vi "Add State to Macro.vi"(5 "Before or After? (Before)":T1, 7 "Before (or After) State":string, 8 "error in (no error)":errorcluster, 9 "State to Add":string, 10 "Macro Name":string, 11 "JKI SM in":refnum<class "JKI SM.lvclass">) -> (0 "error out":errorcluster, 3 "JKI SM out":refnum<class "JKI SM.lvclass">)   [LabVIEW 2013, in "JKI State Machine API.lvlib" / "JKI SM.lvclass"]
uses:
  JKI SM.lvclass
  Typedefs/Before or After -- Enum.ctl
  JKI SM.lvclass/JKI SM.ctl
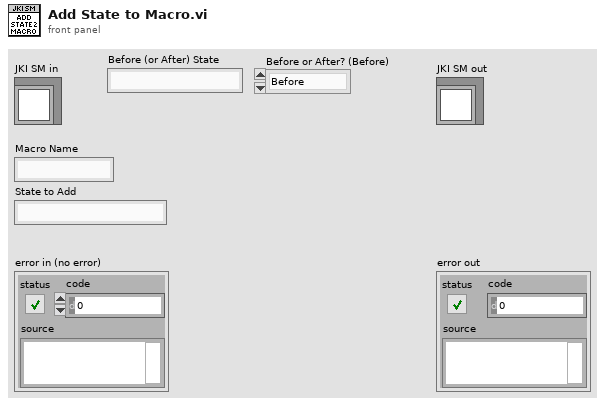
[diagram p1: front panel]
types:
  T1 = typedef "Before or After -- Enum.ctl" = enum16{"Before", "After"}
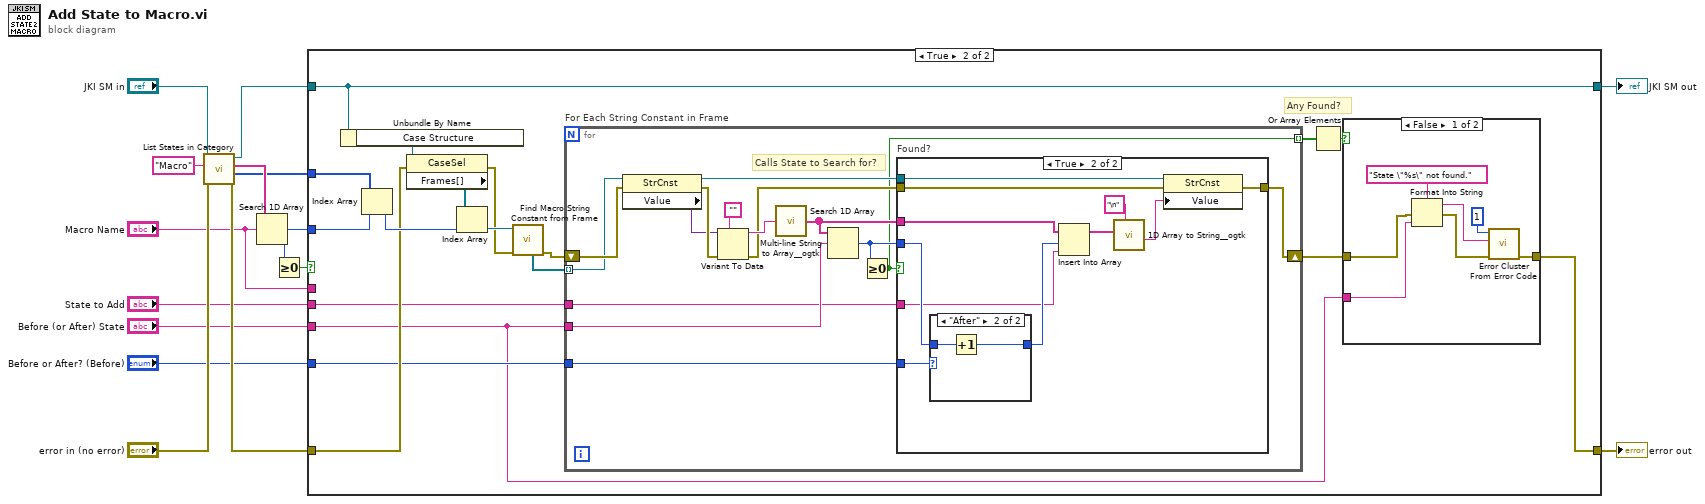
[diagram p0: block diagram]
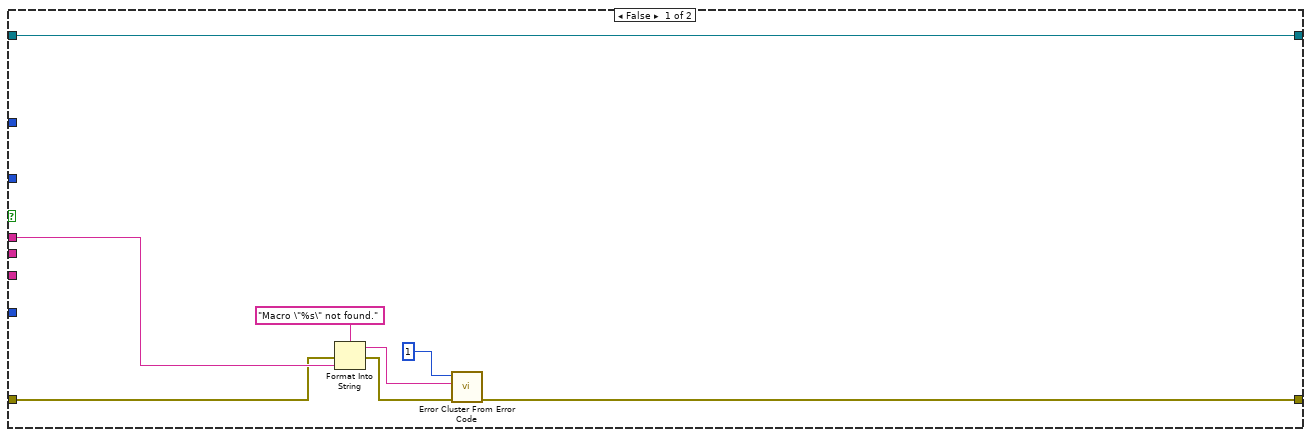
[diagram p2: hidden frame]
diagram:
  n1 = call "List States in Category.vi"("error in (no error)"="error in (no error)", "Category"="Macro", "JKI SM in"="JKI SM in") -> ("error out"=w12:errorcluster, "State Frame Indices"=w13:i32[], "States"=w14:string[], "JKI SM out"=w5:refnum<class "JKI SM.lvclass">)  [unwired: 4 in, 1 out]
  n2 = Search 1D Array(1D array=w14, element="Macro Name") -> (index of element=w3:i32)  [unwired: 1 in]
  n3 = Greater Or Equal To 0?(x=w3) -> (x >= 0?=w4:bool)
  n4 = case shown="True" w4 {
    tunnel: w13 -> [_ w41]
    tunnel: w3 -> [_ w40]
    tunnel: w12 -> [w17 w35]
    tunnel: [w22 w26] -> w9
    tunnel: "Before or After? (Before)" -> [_ w31]
    tunnel: "Before (or After) State" -> [_ w24]
    tunnel: "State to Add" -> [_ w30]
    tunnel: w5 -> [w23 w29]
    tunnel: [w23 w29] -> w2
    tunnel: "Macro Name" -> [w20 _]
    frame False {
      n5 = Format Into String(format string="Macro \"%s\" not found.", error in=w17, w20) -> (resulting string=w19:string, error out=w16:errorcluster)  [unwired: 1 in]
      n6 = call <vilib>:"Error Cluster From Error Code.vi"("error in (no error)"=w16, "error message (\"\")"=w19, "error code (0)"=1) -> ("error out"=w22:errorcluster)  [unwired: 6 in]
    }
    frame True {
      # "Any Found?"
      n7 = Unbundle By Name(w29) -> ("Case Structure"=w39:refnum<vi>)
      n8 = Index Array(array=w41, index=w40) -> (element=w38:i32)
      n9 = property class="CaseSel"(reference=w39, error in=w35) -> (error out=w36:errorcluster, "Frames[]"=w33:refnum<vi>[])  [unwired: 1 out]
      n10 = Index Array(array=w33, index=w38) -> (element=w37:refnum<vi>)
      n11 = call "Find Macro String Constant from Frame.vi"("error in (no error)"=w36, "Diagram in"=w37) -> ("error out"=w34:errorcluster, "All String Constants"=w32:refnum<vi>[])  [unwired: 6 in, 2 out]
      n12 = for "For Each String Constant in Frame" {
        tunnel: w32 -> [w60] mode=indexing
        shift-right: [w51] -> w25
        shift-left: w34 -> [w64]
        tunnel: w31 -> [w57]
        tunnel: w24 -> [w56]
        tunnel: w30 -> [w55]
        tunnel: [w50] -> w28 mode=indexing
        # "Calls State to Search for?"
        n13 = property class="StrCnst"(reference=w60, error in=w64) -> (reference out=w53:refnum<vi>, error out=w63:errorcluster, "Value"=w61:variant)
        n14 = Variant To Data(error in=w63, type="", Variant=w61) -> (data=w58:string, error out=w52:errorcluster)
        n15 = call <userlib>:"Multi-line String to Array__ogtk.vi"("string"=w58) -> ("lines"=w59:string[])
        n16 = Search 1D Array(1D array=w59, element=w56) -> (index of element=w54:i32)  [unwired: 1 in]
        n17 = Greater Or Equal To 0?(x=w54) -> (x >= 0?=w50:bool)
        n18 = case "Found?" shown="True" w50 {
          tunnel: w54 -> [_ w76]
          tunnel: w59 -> [_ w74]
          tunnel: w57 -> [_ w71]
          tunnel: w55 -> [_ w70]
          tunnel: w53 -> [_ w69]
          tunnel: w52 -> [w65 w67]
          tunnel: [w65 w66] -> w51
          frame False {
          }
          frame True {
            n19 = case shown="\"After\"" w71 {
              tunnel: [w77 w79] -> w75
              tunnel: w76 -> [w77 w78]
              frame "Before" {
              }
              frame "After" {
                n20 = Increment(x=w78) -> (x+1=w79:i32)
              }
            }
            n21 = Insert Into Array(array=w74, index=w75, new element=w70) -> (w73:string[])
            n22 = call <userlib>:"1D Array to String__ogtk.vi"("delimiter (Tab)"="\n", "Array of Strings"=w73) -> ("delimited string"=w68:string)  [unwired: 9 in]
            n23 = property class="StrCnst"(reference=w69, error in=w67, "Value"=w68) -> (error out=w66:errorcluster)  [unwired: 1 out]
          }
        }
      }
      n24 = Or Array Elements(Boolean array=w28) -> (logical OR=w27:bool)
      n25 = case shown="False" w27 {
        tunnel: [w44 w49] -> w26
        tunnel: w25 -> [w43 w49]
        tunnel: w24 -> [w42 _]
        frame False {
          n26 = Format Into String(format string="State \"%s\" not found.", error in=w43, w42) -> (resulting string=w46:string, error out=w48:errorcluster)  [unwired: 1 in]
          n27 = call <vilib>:"Error Cluster From Error Code.vi"("error in (no error)"=w48, "error message (\"\")"=w46, "error code (0)"=1) -> ("error out"=w44:errorcluster)  [unwired: 6 in]
        }
        frame True {
        }
      }
    }
  }
  "error out" <- w9
  "JKI SM out" <- w2
